vi "Fit Transform.vi"(7 "Type X":T1(ring), 8 "error in (no error)":errorcluster caption="entrée d'erreur (pas d'erreur)", 9 "y":string[][](array[string]), 10 "X":string[][](array[string]), 11 "FeatureHasher.lvclass":refnum<class "FeatureHasher.lvclass">) -> (0 "error out":errorcluster caption="sortie d'erreur", 2 "Data":T2, 3 "FeatureHasher.lvclass":refnum<class "FeatureHasher.lvclass">)   [LabVIEW 2020, in "FeatureHasher.lvclass"]
doc: "Fit to data, then transform it.\n\nFits transformer to X and y with optional parameters fit_params and returns a transformed version of X.\n\nReturns : \n\n- X_new : ndarray array of shape (n_samples, n_features_new)\nTransformed array."
uses:
  FeatureHasher.lvclass
  FeatureHasher.lvclass/FeatureHasher.ctl
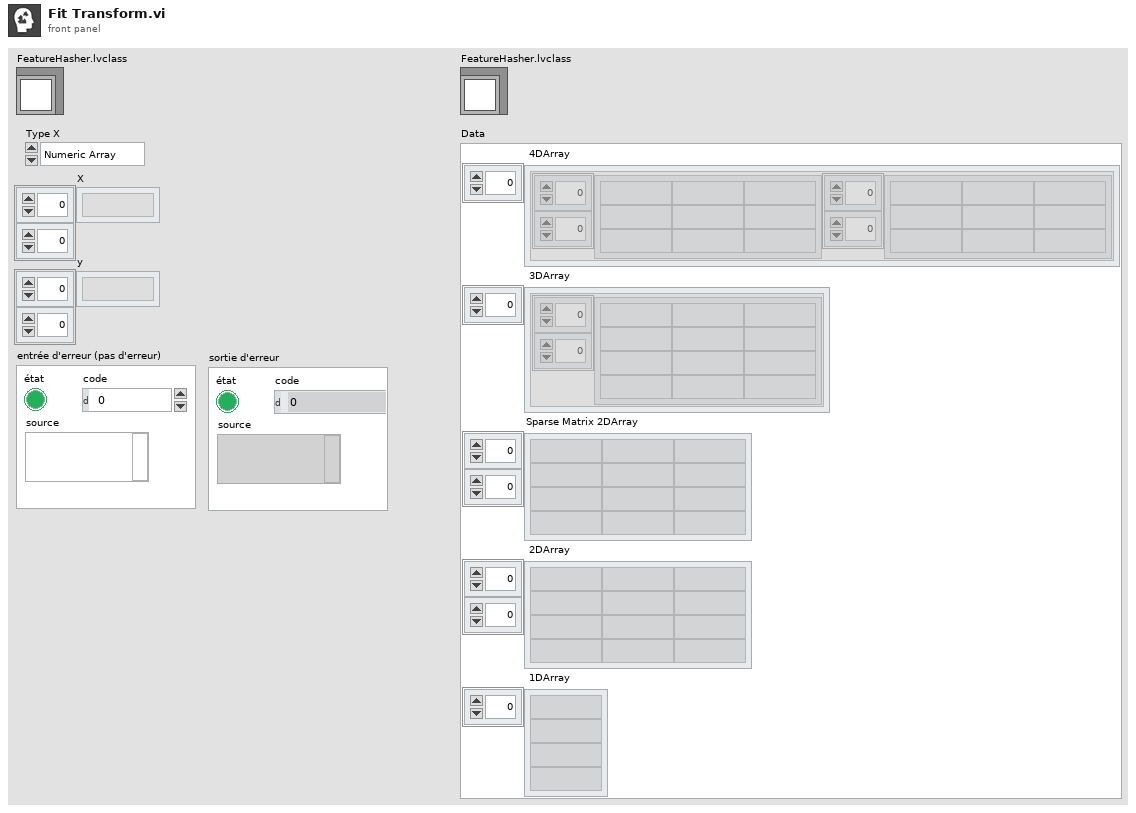
[diagram p1: front panel]
types:
  T1 = enum16{"Numeric Array", "String Array", "Sparse"}
  T2 = cluster{" 4DArray":cluster{"1":string[][], "2":string[][]}[], " 3DArray":cluster{"Tableau":string[][]}[], "Sparse Matrix 2DArray":string[][], " 2DArray":string[][], " 1DArray":string[]}
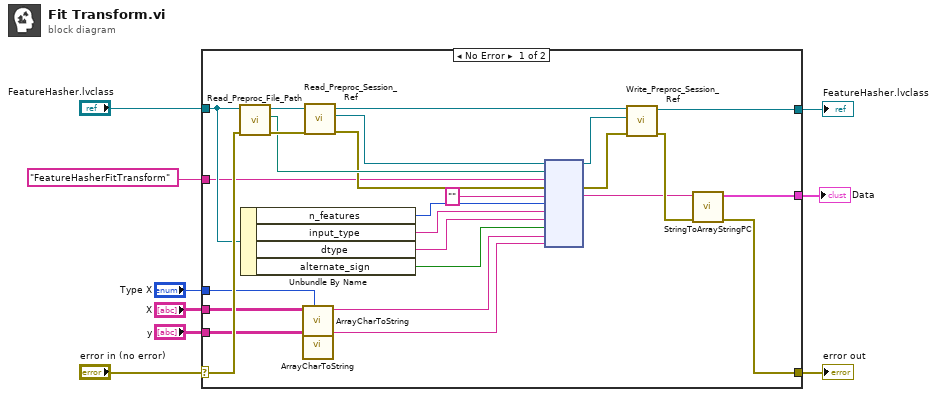
[diagram p0: block diagram]
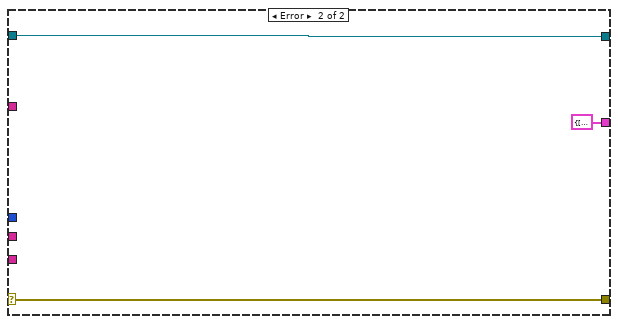
[diagram p2: hidden frame]
diagram:
  n1 = case shown="No Error" "error in (no error)" {
    selector: "error in (no error)" -> [w23 w38]
    tunnel: [w11 w38] -> w8
    tunnel: [w19 w37] -> w6
    tunnel: "FeatureHasher.lvclass" -> [w22 w37]
    tunnel: "FeatureHasherFitTransform" ("Fonction") -> [w21 _]
    tunnel: "X" -> [w18 _]
    tunnel: [w10 T2 {" 4DArray"=[], " 3DArray"=[], "Sparse Matrix 2DArray"=[], " 2DArray"=[], " 1DArray"=[]} ("Data")] -> w1
    tunnel: "y" -> [w15 _]
    tunnel: "Type X" -> [w17 _]
    frame No Error {
      n2 = call-dynamic "Read_Preproc_File_Path.vi"("error in (no error)"=w23, "Python in"=w22) -> ("error out"=w34:errorcluster, "File_Path"=w33:path, "Python out"=w35:refnum<class "FeatureHasher.lvclass">)  [unwired: 7 in]
      n3 = Unbundle By Name(w22) -> ("n_features"=w26:i32, "input_type"=w25:string, "dtype"=w24:string, "alternate_sign"=w20:bool)
      n4 = call "ArrayCharToString.vi"("Type"=w17, "TAB"=w18) -> ("Instruction"=w16:string)  [unwired: 9 in]
      n5 = call "ArrayCharToString.vi"("TAB"=w15) -> ("Instruction"=w14:string)  [unwired: 10 in]
      n6 = call-dynamic "Read_Preproc_Session_Ref.vi"("error in (no error)"=w34, "Python in"=w35) -> ("error out"=w31:errorcluster, "Session_ref"=w32:refnum<k35>, "Python out"=w30:refnum<class "FeatureHasher.lvclass">)  [unwired: 7 in]
      n7 = node(w32, w33, w21, w31, "", w26, w25, w24, w20, w16, w14) -> (w28:refnum<k35>, w29:errorcluster, w12:string)  [unwired: 6 in, 2 out]
      n8 = call-dynamic "Write_Preproc_Session_Ref.vi"("error in (no error)"=w29, "Session_ref"=w28, "Python in"=w30) -> ("error out"=w13:errorcluster, "Python out"=w19:refnum<class "FeatureHasher.lvclass">)  [unwired: 7 in]
      n9 = call "StringToArrayStringPC.vi"("sortie d'erreur"=w13, "Return value"=w12) -> ("sortie d'erreur"=w11:errorcluster, "Data"=w10:T2)  [unwired: 8 in]
    }
    frame Error {
    }
  }
  "error out" <- w8
  "FeatureHasher.lvclass" <- w6
  "Data" <- w1
